vi "Place Number to Proper Engl Text.vi"(5 "Numeric":ext) -> (1 "String":string)   [LabVIEW 2009]
doc: "Converts a place number to proper English text (examples: 1 becomes first, 15 becoms fifteenth). Rounds off to whole numbers and can handle up to 10^63 (vigintillion) places."
panel:
  out "hasOnesPlace":bool
  out "isTeen":bool
  out "hasTensPlace":bool
  out "hasHundredsPlace":bool
  # "[OpenG VI Tags] ***Do Not Remove***"
  # "Place Number to Proper English Text.vi\n\nConverts a place integer to proper English text.\n\nPlease visit http://www.OpenG.org to learn about the\nOpen Source LabVIEW software movement.\n\nNOTICE -- YOU MUST LEAVE THIS NOTICE IN PLACE.  PER THE TERMS OF THE LICENSE BELOW, YOU MAY SUBLICENSE THIS SOFTWARE \nIN ANY WAY THAT DOES NOT CONFLICT WITH THIS LICENSE.\n\n### BSD License (http://www.opensource.org/licenses/bsd-license.php) Begin ###\n \nCopyright (c) 2002, Jim Kring <jim@jimkring.com>\nCopyright (c) 2006, MKS Instruments, Inc., author: Doug Femec<doug_femec@mksinst.com>, IM dafemec\n\nAll rights reserved.\n\nRedistribution and use in source and binary forms, with or without modification, are permitted provided that the following conditions are met:\n\n    * Redistributions of source code must retain the above copyright notice, this list of conditions and the following disclaimer.\n    * Redistributions in binary form must reproduce the above copyright notice, this list of conditions and the following disclaimer in the \n       documentation and/or other materials provided with the distribution.\n    * Neither the name of SciWare, James Kring, Inc., nor the names of its contributors may be used to endorse or promote products derived \n       from this software without specific prior written permission.\n\nTHIS SOFTWARE IS PROVIDED BY THE COPYRIGHT HOLDERS AND CONTRIBUTORS \"AS IS\" AND ANY EXPRESS OR IMPLIED WARRANTIES, \nINCLUDING, BUT NOT LIMITED TO, THE IMPLIED WARRANTIES OF MERCHANTABILITY AND FITNESS FOR A PARTICULAR PURPOSE ARE \nDISCLAIMED. IN NO EVENT SHALL THE COPYRIGHT OWNER OR CONTRIBUTORS BE LIABLE FOR ANY DIRECT, INDIRECT, INCIDENTAL,\n SPECIAL, EXEMPLARY, OR CONSEQUENTIAL DAMAGES (INCLUDING, BUT NOT LIMITED TO, PROCUREMENT OF SUBSTITUTE GOODS OR \nSERVICES; LOSS OF USE, DATA, OR PROFITS; OR BUSINESS INTERRUPTION) HOWEVER CAUSED AND ON ANY THEORY OF LIABILITY, \nWHETHER IN CONTRACT, STRICT LIABILITY, OR TORT (INCLUDING NEGLIGENCE OR OTHERWISE) ARISING IN ANY WAY OUT OF THE USE \nOF THIS SOFTWARE, EVEN IF ADVISED OF THE POSSIBILITY OF SUCH DAMAGE.\n\n### BSD License End ###"
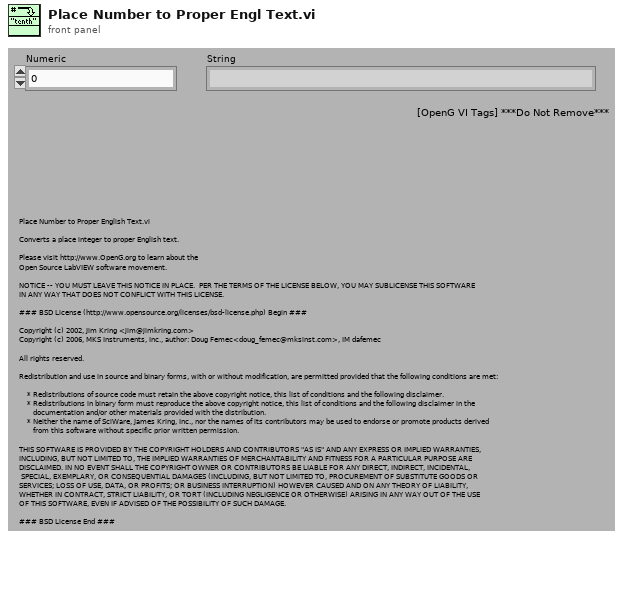
[diagram p1: front panel]
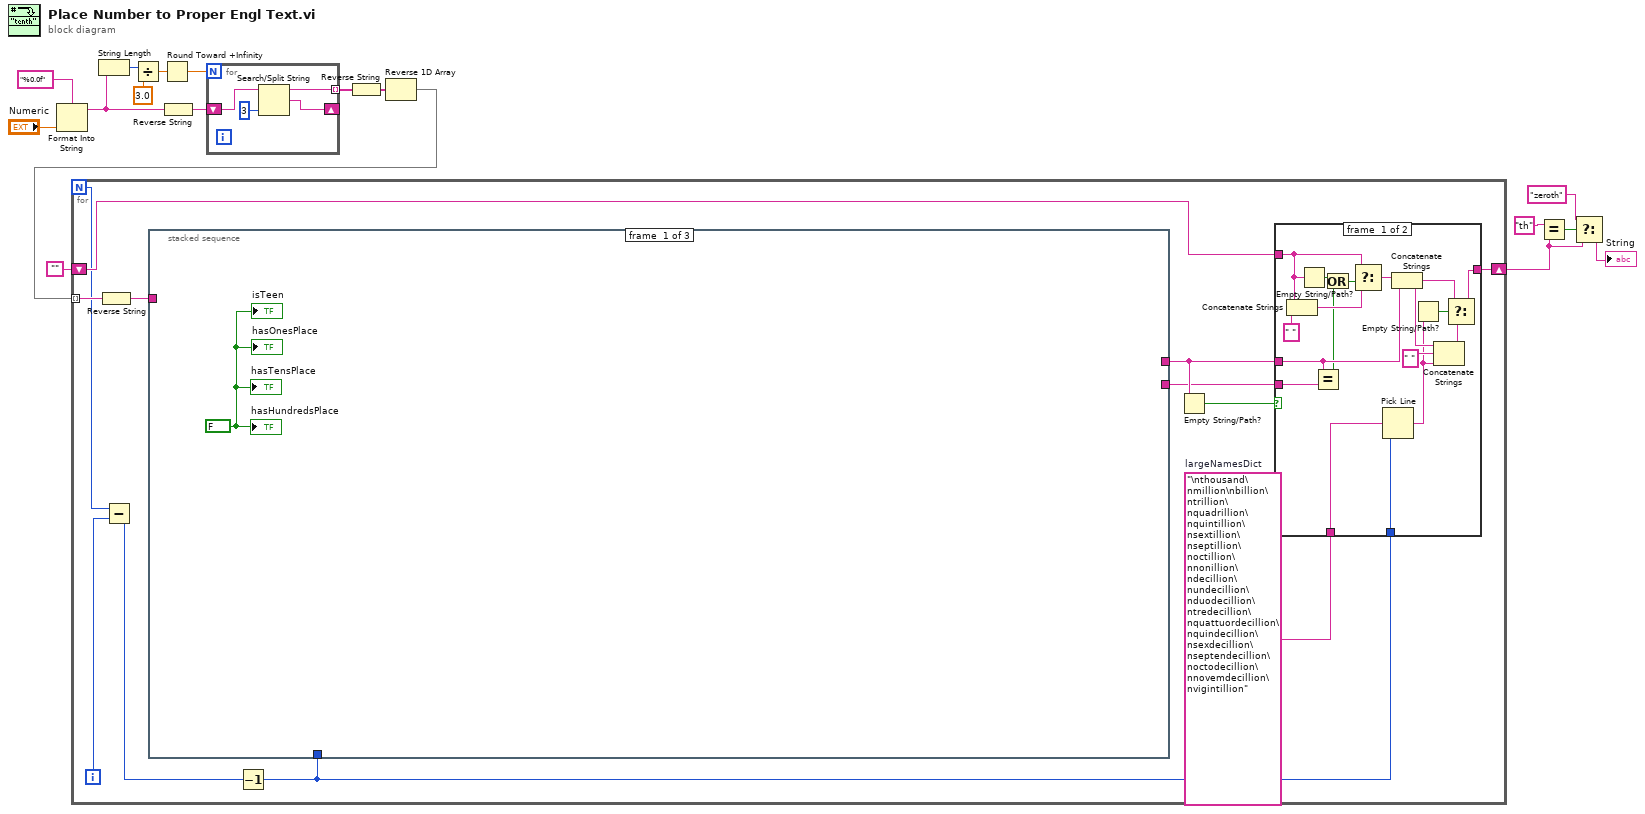
[diagram p0: block diagram]
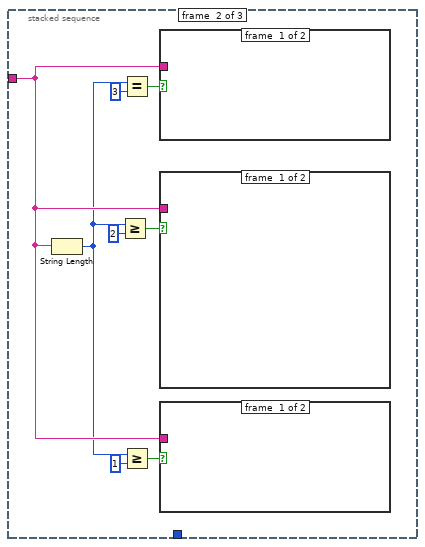
[diagram p3: hidden frame]
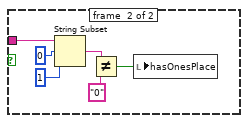
[diagram p4: hidden frame]
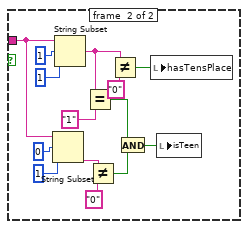
[diagram p5: hidden frame]
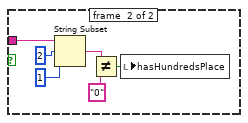
[diagram p6: hidden frame]
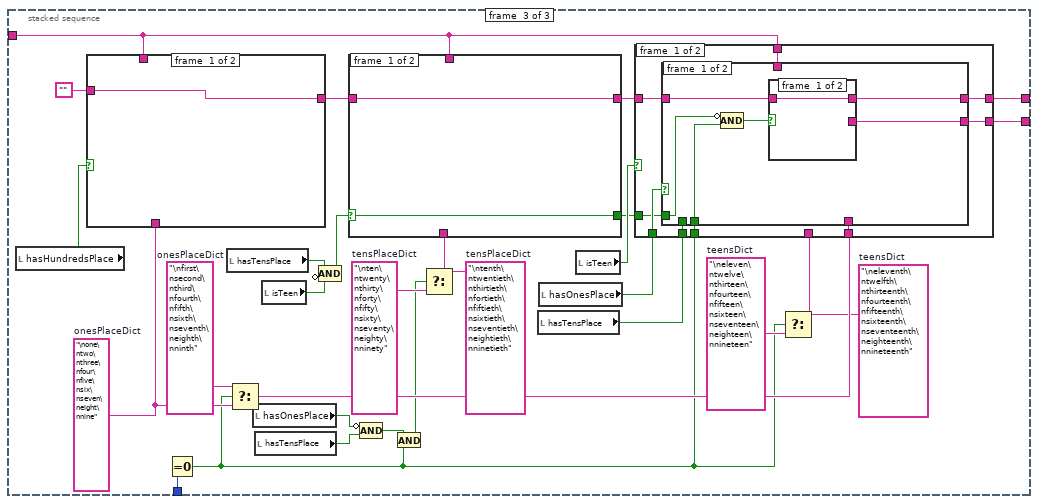
[diagram p7: hidden frame]
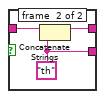
[diagram p8: hidden frame]
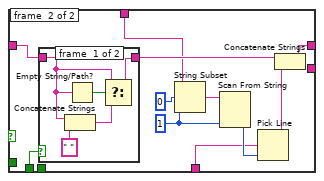
[diagram p9: hidden frame]
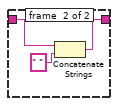
[diagram p10: hidden frame]
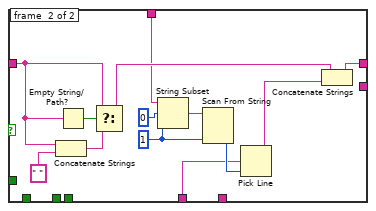
[diagram p11: hidden frame]
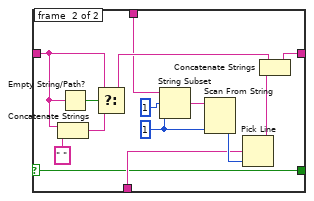
[diagram p12: hidden frame]
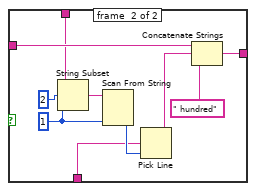
[diagram p13: hidden frame]
diagram:
  n1 = Format Into String(format string="%0.0f" ("Format String"), "Numeric") -> (resulting string=w12:string)  [unwired: 2 in, 1 out]
  n2 = String Length(string=w12) -> (length=w15:i32)
  n3 = Divide(x=w15, y=3.0) -> (x/y=w14:dbl)
  n4 = Round Toward +Infinity(x=w14) -> (ceil(x): smallest int >= x=w13:dbl)
  n5 = Reverse String(1:w12) -> (0:w11:string)
  n6 = for {
    N: w13 -> [_]
    shift-right: [w19] -> _
    shift-left: w11 -> [w21]
    tunnel: [w18] -> w10 mode=indexing
    n7 = Search/Split String(string=w21, offset (0)=3) -> (substring before match=w18:string, match + rest of string=w19:string)  [unwired: 1 in, 1 out]
  }
  n8 = Reverse String(1:w10) -> (0:w8:string[])
  n9 = Reverse 1D Array(array=w8) -> (reversed array=w7:string[])
  n10 = for {
    N -> [w27]
    shift-right: [w28] -> w4
    shift-left: "" -> [w29]
    tunnel: w7 -> [w32] mode=indexing
    i -> [w25]
    w24 = "\nthousand\nmillion\nbillion\ntrillion\nquadrillion\nquintillion\nsextillion\nseptillion\noctillion\nnonillion\ndecillion\nundecillion\nduodecillion\ntredecillion\nquattuordecillion\nquindecillion\nsexdecillion\nseptendecillion\noctodecillion\nnovemdecillion\nvigintillion"  # largeNamesDict
    n11 = Reverse String(1:w32) -> (0:w33:string)
    n12 = Subtract(x=w27, y=w25) -> (x-y=w26:i32)
    n13 = Decrement(x=w26) -> (x-1=w22:i32)
    n14 = stacked-sequence {
      tunnel: w33 -> [_ w54 w104]
      tunnel: [_ _ w105] -> w30
      tunnel: [_ _ w103] -> w23
      tunnel: w22 -> [_ _ w99]
      frame #0 {
        w52 = FALSE
        "hasOnesPlace" <- w52
        "isTeen" <- w52
        "hasTensPlace" <- w52
        "hasHundredsPlace" <- w52
      }
      frame #1 {
        n15 = String Length(string=w54) -> (length=w53:i32)
        n16 = Greater Or Equal?(x=w53, y=2) -> (x >= y?=w57:bool)
        n17 = Equal?(x=w53, y=3) -> (x = y?=w59:bool)
        n18 = Greater Or Equal?(x=w53, y=1) -> (x >= y?=w56:bool)
        n19 = case shown="False" w59 {
          tunnel: w54 -> [_ w81]
          frame #0 {
          }
          frame #1 {
            n20 = String Subset(string=w81, offset (0)=2, length (rest)=1 ("length (rest)")) -> (substring=w84:string)
            n21 = Not Equal?(x=w84, y="0") -> (x != y?=w86:bool)
            n22 = local write "hasHundredsPlace"(w86) -> ()
          }
        }
        n23 = case shown="True" w57 {
          tunnel: w54 -> [_ w76]
          frame #0 {
          }
          frame #1 {
            n24 = String Subset(string=w76, offset (0)=0, length (rest)=1 ("length (rest)")) -> (substring=w74:string)
            n25 = String Subset(string=w76, offset (0)=1, length (rest)=1 ("length (rest)")) -> (substring=w72:string)
            n26 = Equal?(x=w72, y="1") -> (x = y?=w71:bool)
            n27 = Not Equal?(x=w74, y="0") -> (x != y?=w73:bool)
            n28 = Not Equal?(x=w72, y="0") -> (x != y?=w70:bool)
            n29 = And(x=w71, y=w73) -> (x .and. y?=w69:bool)
            n30 = local write "hasTensPlace"(w70) -> ()
            n31 = local write "isTeen"(w69) -> ()
          }
        }
        n32 = case shown="True" w56 {
          tunnel: w54 -> [_ w61]
          frame #0 {
          }
          frame #1 {
            n33 = String Subset(string=w61, offset (0)=0, length (rest)=1 ("length (rest)")) -> (substring=w64:string)
            n34 = Not Equal?(x=w64, y="0") -> (x != y?=w66:bool)
            n35 = local write "hasOnesPlace"(w66) -> ()
          }
        }
      }
      frame #2 {
        w100 = "\nfirst\nsecond\nthird\nfourth\nfifth\nsixth\nseventh\neighth\nninth"  # onesPlaceDict
        w92 = "\ntenth\ntwentieth\nthirtieth\nfortieth\nfiftieth\nsixtieth\nseventieth\neightieth\nninetieth"  # tensPlaceDict
        w96 = "\neleventh\ntwelfth\nthirteenth\nfourteenth\nfifteenth\nsixteenth\nseventeenth\neighteenth\nnineteenth"  # teensDict
        w97 = "\neleven\ntwelve\nthirteen\nfourteen\nfifteen\nsixteen\nseventeen\neighteen\nnineteen"  # teensDict
        w94 = "\nten\ntwenty\nthirty\nforty\nfifty\nsixty\nseventy\neighty\nninety"  # tensPlaceDict
        w101 = "\none\ntwo\nthree\nfour\nfive\nsix\nseven\neight\nnine"  # onesPlaceDict
        n36 = local read "hasHundredsPlace"() -> (w115:bool)
        n37 = case shown="False" w115 {
          tunnel: "" -> [w183 w186]
          tunnel: [w183 w187] -> w110
          tunnel: w104 -> [_ w185]
          tunnel: w101 -> [_ w184]
          frame #0 {
          }
          frame #1 {
            w191 = 1 ("length (rest)")
            n38 = String Subset(string=w185, offset (0)=2, length (rest)=w191) -> (substring=w192:string)
            n39 = Scan From String(input string=w192, default 1=w191) -> (output 1=w190:i32)  [unwired: 3 in, 3 out]
            n40 = Pick Line(multi-line string=w184, line index=w190) -> (output string=w188:string)  [unwired: 1 in]
            n41 = Concatenate Strings(w186, w188, " hundred" ("Substring")) -> (w187:string)
          }
        }
        n42 = Equal To 0?(x=w99) -> (x = 0?=w93:bool)
        n43 = local read "hasTensPlace"() -> (w112:bool)
        n44 = Select(t=w100, s=w93, f=w101) -> (s? t:f=w102:string)
        n45 = local read "hasOnesPlace"() -> (w89:bool)
        n46 = local read "hasTensPlace"() -> (w88:bool)
        n47 = local read "isTeen"() -> (w113:bool)
        n48 = Compound Arithmetic op=AND(w112, invert w113) -> (w111:bool)
        n49 = Compound Arithmetic op=AND(invert w89, w88) -> (w87:bool)
        n50 = And(x=w87, y=w93) -> (x .and. y?=w90:bool)
        n51 = Select(t=w92, s=w90, f=w94) -> (s? t:f=w95:string)
        n52 = case shown="True" w111 {
          selector: w111 -> [w167 w169]
          tunnel: w110 -> [w168 w172]
          tunnel: [w168 w174] -> w109
          tunnel: w104 -> [_ w171]
          tunnel: w95 -> [_ w170]
          tunnel: [w167 w169] -> w91
          frame #0 {
          }
          frame #1 {
            w178 = 1 ("length (rest)")
            n53 = Concatenate Strings(w172, " " ("Substring")) -> (w180:string)
            n54 = Empty String/Path?(string/path=w172) -> (empty?=w182:bool)
            n55 = Select(t=w172, s=w182, f=w180) -> (s? t:f=w173:string)
            n56 = String Subset(string=w171, offset (0)=1, length (rest)=w178) -> (substring=w177:string)
            n57 = Scan From String(input string=w177, default 1=w178) -> (output 1=w179:i32)  [unwired: 3 in, 3 out]
            n58 = Pick Line(multi-line string=w170, line index=w179) -> (output string=w175:string)  [unwired: 1 in]
            n59 = Concatenate Strings(w173, w175) -> (w174:string)
          }
        }
        n60 = local read "hasTensPlace"() -> (w106:bool)
        n61 = local read "hasOnesPlace"() -> (w107:bool)
        n62 = local read "isTeen"() -> (w108:bool)
        n63 = Select(t=w96, s=w93, f=w97) -> (s? t:f=w98:string)
        n64 = case shown="False" w108 {
          tunnel: w109 -> [w123 w156]
          tunnel: [w121 w158] -> w105
          tunnel: w107 -> [w124 _]
          tunnel: w106 -> [w122 _]
          tunnel: w104 -> [w120 w155]
          tunnel: w102 -> [w119 _]
          tunnel: w98 -> [_ w154]
          tunnel: [w118 _] -> w103
          tunnel: w93 -> [w117 _]
          tunnel: w91 -> [w116 _]
          frame #0 {
            n65 = case shown="True" w124 {
              tunnel: w123 -> [w130 w144]
              tunnel: w122 -> [_ w145]
              tunnel: [w129 w137] -> w121
              tunnel: w120 -> [_ w136]
              tunnel: w119 -> [_ w135]
              tunnel: [w128 _] -> w118
              tunnel: w117 -> [w127 _]
              tunnel: w116 -> [w125 _]
              frame #0 {
                n66 = Compound Arithmetic op=AND(invert w125, w127) -> (w126:bool)
                n67 = case shown="True" w126 {
                  tunnel: w130 -> [w131 w134]
                  tunnel: [w131 w133] -> w129
                  tunnel: [_ w132] -> w128
                  frame #0 {
                  }
                  frame #1 {
                    w132 = "th" ("string")
                    n68 = Concatenate Strings(w134, w132) -> (w133:string)
                  }
                }
              }
              frame #1 {
                w142 = 1 ("length (rest)")
                n69 = case shown="True" w145 {
                  tunnel: w144 -> [w147 w153]
                  tunnel: [w146 w151] -> w138
                  frame #0 {
                    n70 = Concatenate Strings(w147, " " ("Substring")) -> (w150:string)
                    n71 = Empty String/Path?(string/path=w147) -> (empty?=w148:bool)
                    n72 = Select(t=w147, s=w148, f=w150) -> (s? t:f=w146:string)
                  }
                  frame #1 {
                    n73 = Concatenate Strings(w153, " " ("Substring")) -> (w151:string)
                  }
                }
                n74 = String Subset(string=w136, offset (0)=0, length (rest)=w142) -> (substring=w141:string)
                n75 = Scan From String(input string=w141, default 1=w142) -> (output 1=w143:i32)  [unwired: 3 in, 3 out]
                n76 = Pick Line(multi-line string=w135, line index=w143) -> (output string=w139:string)  [unwired: 1 in]
                n77 = Concatenate Strings(w138, w139) -> (w137:string)
              }
            }
          }
          frame #1 {
            w162 = 1 ("length (rest)")
            n78 = Concatenate Strings(w156, " " ("Substring")) -> (w164:string)
            n79 = Empty String/Path?(string/path=w156) -> (empty?=w166:bool)
            n80 = Select(t=w156, s=w166, f=w164) -> (s? t:f=w157:string)
            n81 = String Subset(string=w155, offset (0)=0, length (rest)=w162) -> (substring=w161:string)
            n82 = Scan From String(input string=w161, default 1=w162) -> (output 1=w163:i32)  [unwired: 3 in, 3 out]
            n83 = Pick Line(multi-line string=w154, line index=w163) -> (output string=w159:string)  [unwired: 1 in]
            n84 = Concatenate Strings(w157, w159) -> (w158:string)
          }
        }
      }
    }
    n85 = Empty String/Path?(string/path=w30) -> (empty?=w31:bool)
    n86 = case shown="False" w31 {
      tunnel: w30 -> [w36 _]
      tunnel: w29 -> [w47 w51]
      tunnel: [w44 w51] -> w28
      tunnel: w22 -> [w39 _]
      tunnel: w24 -> [w38 _]
      tunnel: w23 -> [w37 _]
      frame #0 {
        n87 = Concatenate Strings(w47, " " ("Substring")) -> (w48:string)
        n88 = Empty String/Path?(string/path=w47) -> (empty?=w50:bool)
        n89 = Equal?(x=w36, y=w37) -> (x = y?=w35:bool)
        n90 = Or(x=w50, y=w35) -> (x .or. y?=w34:bool)
        n91 = Select(t=w47, s=w34, f=w48) -> (s? t:f=w46:string)
        n92 = Pick Line(multi-line string=w38, line index=w39) -> (output string=w41:string)  [unwired: 1 in]
        n93 = Concatenate Strings(w46, w36) -> (w42:string)
        n94 = Empty String/Path?(string/path=w41) -> (empty?=w45:bool)
        n95 = Concatenate Strings(w42, " " ("Substring"), w41) -> (w40:string)
        n96 = Select(t=w42, s=w45, f=w40) -> (s? t:f=w44:string)
      }
      frame #1 {
      }
    }
  }
  n97 = Equal?(x="th", y=w4) -> (x = y?=w5:bool)
  n98 = Select(t="zeroth", s=w5, f=w4) -> (s? t:f=→"String":string)
